vi "Read Work URL as Path.vi"(11 "ViewableActor in":refnum<class "ViewableActor.lvclass">) -> (2 "Path":path, 3 "ViewableActor out":refnum<class "ViewableActor.lvclass">)   [LabVIEW 2020, in "ViewableActor.lvlib" / "ViewableActor.lvclass"]
uses:
  ViewableActor.lvclass
  ViewableActor.lvclass/ViewableActor.ctl
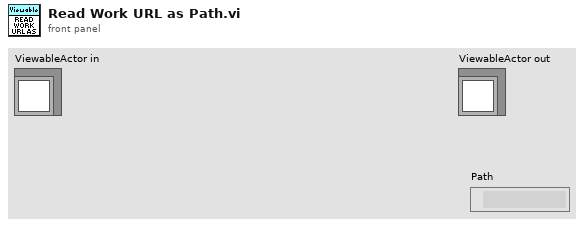
[diagram p1: front panel]
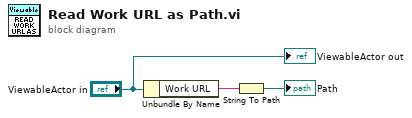
[diagram p0: block diagram]
diagram:
  n1 = Unbundle By Name("ViewableActor in") -> ("Work URL"=w2:string)
  n2 = String To Path(string=w2) -> (path=→"Path":path)
  "ViewableActor out" <- "ViewableActor in"
